vi "Gauss Mod Sine Generation.vi"() -> ()   [LabVIEW 2023]
doc: "This example shows the Gaussian Modulated Sine Pattern VI and its envelopes. The envelopes are Gaussian signals."
uses:
  <vilib>/Analysis/1siggen.llb/Ramp Pattern by Samples.vi
  <vilib>/Analysis/1siggen.llb/General Gauss-Mod Sine.vi
  <vilib>/Analysis/NI_AALBase.lvlib
panel:
  out "Gauss-Mod Sine Pattern and its envelopes":cluster{dbl[], dbl[]}[](graph)
  in  "attenuation [dB]":dbl=6.0
  in  "center frequency [Hz]":dbl=1.0
  in  "Normalized bandwidth":dbl=0.15
  in  "delta t [s]":dbl=0.1
  in  "delay [s]":dbl=12.8
  in  "amplitude":dbl=1.0
  in  "samples":i32=256
  # "Overview: Illustrates the use of the Gaussian Modulated Sine Pattern VI.\nRequirements: LabVIEW Full Development System\nInstructions: \n1. Run the VI.\n2. Modify the parameters and run the VI again to view the changes in the graph."
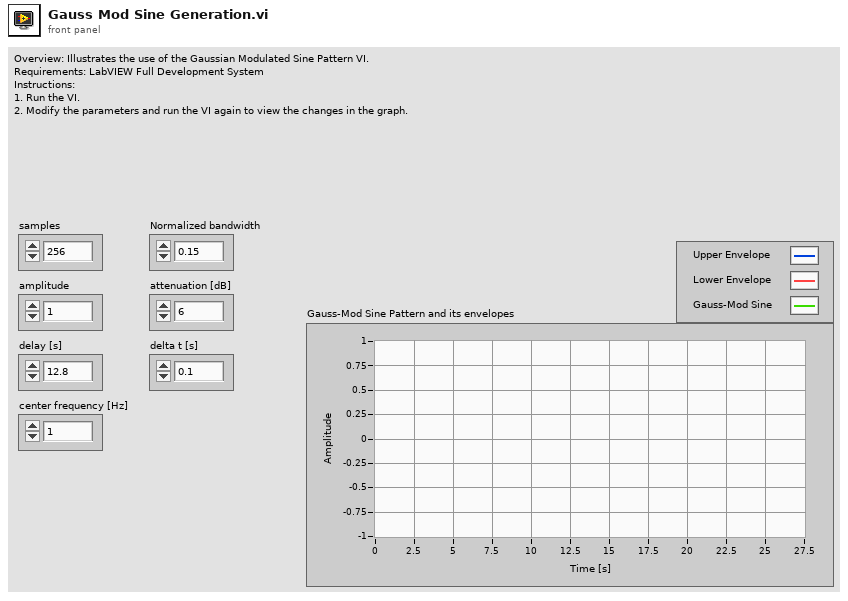
[diagram p1: front panel]
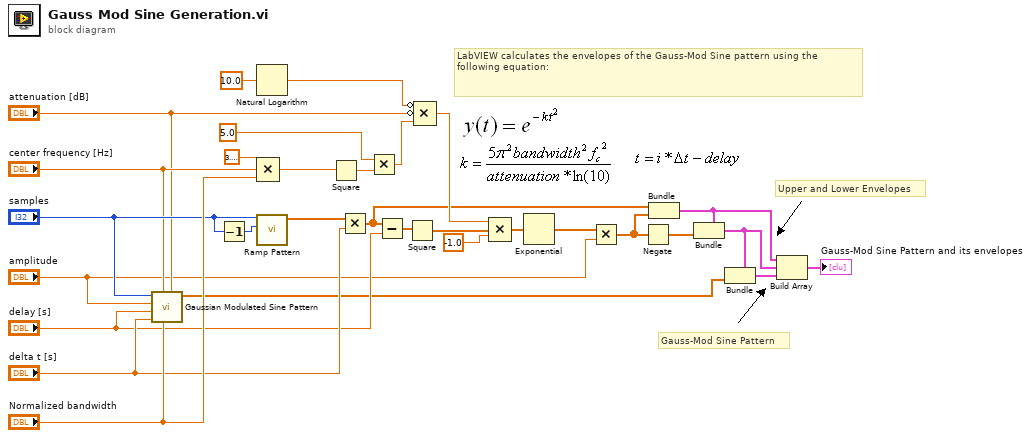
[diagram p0: block diagram]
diagram:
  # "LabVIEW calculates the envelopes of the Gauss-Mod Sine pattern using the following equation:"
  # "Gauss-Mod Sine Pattern"
  # "Upper and Lower Envelopes"
  n1 = call <vilib>:"Gaussian Modulated Sine Pattern.vi"("attenuation (dB)"="attenuation [dB]", "normalized bandwidth"="Normalized bandwidth", "center frequency (Hz)"="center frequency [Hz]", "delta t (s)"="delta t [s]", "delay (s)"="delay [s]", "amplitude"="amplitude", "samples"="samples") -> ("Gauss-Mod Sine Pattern"=w6:dbl[])  [unwired: 3 in, 1 out]
  n2 = Decrement(x="samples") -> (x-1=w29:i32)
  n3 = Natural Logarithm(1:10.0 ("x")) -> (0:w14:dbl)
  n4 = Compound Arithmetic op=MULTIPLY(3.141592653589793, "center frequency [Hz]", "Normalized bandwidth") -> (w21:dbl)
  n5 = call-poly <vilib>:"Ramp Pattern.vi"("end"=w29, "samples"="samples") -> ("Ramp Pattern"=w9:dbl[])  [unwired: 8 in, 1 out]
  n6 = Square(x=w21) -> (x^2=w15:dbl)
  n7 = Multiply(x=w9, y="delta t [s]") -> (x*y=w2:dbl[])
  n8 = Multiply(x=5.0 ("value"), y=w15) -> (x*y=w12:dbl)
  n9 = Subtract(x=w2, y="delay [s]") -> (x-y=w24:dbl[])
  n10 = Square(x=w24) -> (x^2=w23:dbl[])
  n11 = Compound Arithmetic op=MULTIPLY(invert w14, invert "attenuation [dB]", w12) -> (w19:dbl)
  n12 = Compound Arithmetic op=MULTIPLY(w19, w23, -1.0) -> (w22:dbl[])
  n13 = Exponential(1:w22) -> (0:w11:dbl[])
  n14 = Multiply(x=w11, y="amplitude") -> (x*y=w8:dbl[])
  n15 = Negate(x=w8) -> (-x=w7:dbl[])
  n16 = Bundle(w2, w8) -> (w3:cluster{dbl[], dbl[]})  [unwired: 1 in]
  n17 = Bundle(cluster=w3, w7) -> (w4:cluster{dbl[], dbl[]})  [unwired: 1 in]
  n18 = Bundle(cluster=w4, w6) -> (w5:cluster{dbl[], dbl[]})  [unwired: 1 in]
  n19 = Build Array(w3, w4, w5) -> (→"Gauss-Mod Sine Pattern and its envelopes":cluster{dbl[], dbl[]}[])
